vi "Paused Next State.vi"(8 "error in":errorcluster, 11 "Command":T2) -> (0 "error out":errorcluster, 3 "State":T1)   [LabVIEW 2013, in "Standard Engine Runtime.lvclass"]
uses:
  Standard Engine Runtime.lvclass
  Commands.ctl
  <vilib>/NI/Module Execution Interface/Engine Runtime/Execution States.ctl
  <vilib>/NI/Module Execution Interface/Engine Runtime/Engine Runtime Interface.lvclass
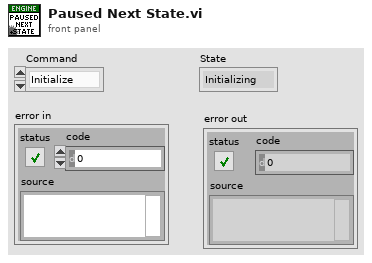
[diagram p1: front panel]
types:
  T1 = typedef "Engine Runtime Interface.lvclass/Execution States.ctl" = enum16{"Initializing", "Paused (Initialized)", "Running", "Set Safe Outputs", "Uninitializing", "Stopped (Uninitialized)", "Error (Uninitialized)", "Safe State (Uninitialized)", "Closed"}
  T2 = typedef "Standard Engine Runtime.lvclass/Commands.ctl" = enum16{"Initialize", "Start", "Pause", "Safe State", "Normal", "Stop", "Shutdown"}
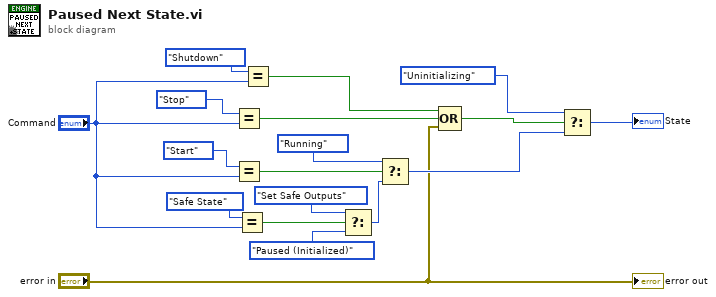
[diagram p0: block diagram]
diagram:
  n1 = Equal?(x=Commands."Stop" ("Commands"), y="Command") -> (x = y?=w13:bool)
  n2 = Equal?(x=Commands."Start" ("Commands"), y="Command") -> (x = y?=w10:bool)
  n3 = Equal?(x=Commands."Safe State" ("Commands"), y="Command") -> (x = y?=w7:bool)
  n4 = Equal?(x=Commands."Shutdown" ("Commands"), y="Command") -> (x = y?=w1:bool)
  n5 = Select(t=Execution_States."Set Safe Outputs", s=w7, f=Execution_States."Paused (Initialized)" ("States")) -> (s? t:f=w5:T1)
  n6 = Select(t=Execution_States."Running" ("States"), s=w10, f=w5) -> (s? t:f=w12:T1)
  n7 = Compound Arithmetic op=OR(w1, w13, "error in") -> (w14:bool)
  n8 = Select(t=Execution_States."Uninitializing" ("States"), s=w14, f=w12) -> (s? t:f=→"State":T1)
  "error out" <- "error in"
